vi "Get BC.vi"(8 "error in (no error)":errorcluster, 10 "Domain":refnum<class "NI_Domain.lvclass">, 11 "BC_Steady_2D_VIRef in":refnum<class "NI_BC_Steady_2D_VIRef.lvclass">) -> (0 "error out":errorcluster, 2 "BC":variant, 3 "BC_Steady_2D_VIRef out":refnum<class "NI_BC_Steady_2D_VIRef.lvclass">)   [LabVIEW 2020, in "NI_PDE.lvlib" / "NI_BC_Steady_2D_VIRef.lvclass"]
uses:
  <vilib>/gmath/pde.llb/BCClass/BC_Steady_2D_VIRef/NI_BC_Steady_2D_VIRef.lvclass
  <vilib>/gmath/pde.llb/DomainClass/NI_Domain.lvclass
  <vilib>/gmath/pde.llb/BCClass/BC_Steady_2D_VIRef/BC Data.ctl
  <vilib>/gmath/pde.llb/Common/PDE_BC Type.ctl
  <vilib>/gmath/pde.llb/Common/PDE_BC Position 2D.ctl
  <vilib>/gmath/pde.llb/BCClass/BC_Steady_2D_VIRef/NI_BC_Steady_2D_VIRef.lvclass/NI_BC_Steady_2D_VIRef.ctl
  <vilib>/gmath/NI_PDE.lvlib
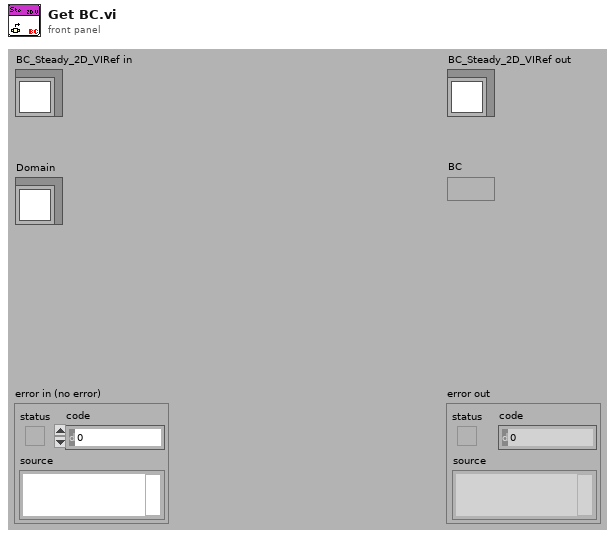
[diagram p1: front panel]
types:
  T1 = typedef "NI_PDE.lvlib/NI_BC_Steady_2D_VIRef.lvclass/BC Data.ctl" = cluster{"type":T2, "position":T3, "G":refnum<vi>, "data":variant}
  T2 = typedef "NI_PDE.lvlib/PDE_BC Type.ctl" = i32
  T3 = typedef "NI_PDE.lvlib/PDE_BC Position 2D.ctl" = i32
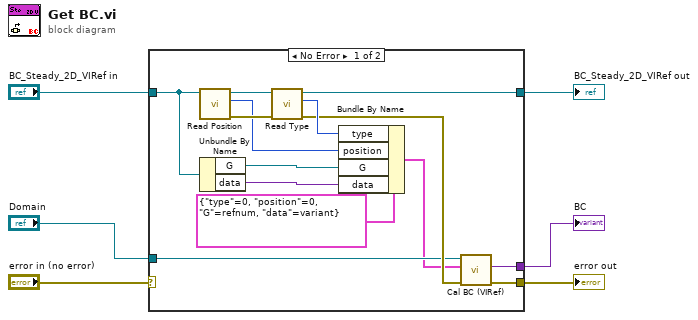
[diagram p0: block diagram]
diagram:
  n1 = case shown="No Error" "error in (no error)" {
    selector: "error in (no error)" -> [_ w22]
    tunnel: "BC_Steady_2D_VIRef in" -> [w13 w21]
    tunnel: "Domain" -> [w10 _]
    tunnel: [w7 _] -> w4
    tunnel: [w19 w21] -> w3
    tunnel: [w9 w22] -> w2
    frame No Error {
      n2 = call-dynamic "Read Position.vi"("BC_Steady_2D.lvclass in"=w13) -> ("error out"=w17:errorcluster, "BC position 2D"=w16:T3, "BC_Steady_2D.lvclass out"=w18:refnum<class "NI_BC_Steady_2D_VIRef.lvclass">)  [unwired: 1 in, 7 out]
      n3 = Unbundle By Name(w13) -> ("G"=w12:refnum<vi>, "data"=w11:variant)
      n4 = call-dynamic "Read Type.vi"("error in (no error)"=w17, "BC.lvclass in"=w18) -> ("error out"=w14:errorcluster, "BC type"=w15:T2, "BC.lvclass out"=w19:refnum<class "NI_BC_Steady_2D_VIRef.lvclass">)  [unwired: 7 out]
      n5 = Bundle By Name(cluster=T1 {"type"=0, "position"=0, "G"=refnum, "data"=variant} ("BC data"), "type"=w15, "position"=w16, "G"=w12, "data"=w11) -> (w8:T1)
      n6 = call-dynamic "Cal BC (VIRef).vi"("error in (no error)"=w14, "BC in"=w8, "Domain in"=w10) -> ("error out"=w9:errorcluster, "BC out"=w7:variant)  [unwired: 7 out]
    }
    frame Error {
    }
  }
  "BC" <- w4
  "error out" <- w2
  "BC_Steady_2D_VIRef out" <- w3
